vi "Throw -8719 error.vi"(7 "window name":string, 8 "error in (no error)":errorcluster, 9 "measurement name":string, 10 "Custom device name":string, 11 "Error":bool) -> (0 "error out":errorcluster)   [LabVIEW 2015, in "Engine Simulation Toolkit System Explorer.lvlib"]
uses:
  Engine Simulation Toolkit System Explorer.lvlib
  <vilib>/Utility/error.llb/Error Cluster From Error Code.vi
  <vilib>/ErrorRing/Error Ring.xnode
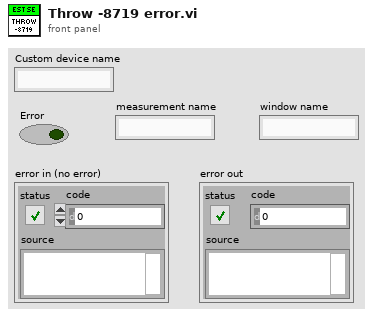
[diagram p1: front panel]
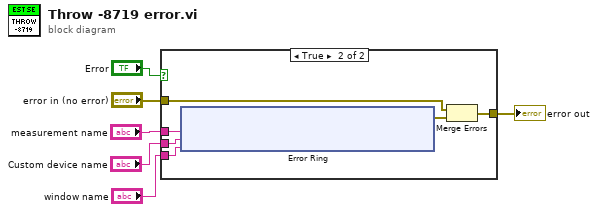
[diagram p0: block diagram]
diagram:
  n1 = case shown="True" "Error" {
    tunnel: "error in (no error)" -> [w7 w13]
    tunnel: "Custom device name" -> [_ w10]
    tunnel: [w7 w11] -> w6
    tunnel: "measurement name" -> [_ w9]
    tunnel: "window name" -> [_ w8]
    frame False {
    }
    frame True {
      n2 = xnode "Error Ring"("parameter 0"=w9, "parameter 1"=w10, "parameter 2"=w8) -> ("error out"=w12:errorcluster)
      n3 = Merge Errors(w13, w12) -> (w11:errorcluster)
    }
  }
  "error out" <- w6
